vi "mqtt_subsriber.vi"() -> ()   [LabVIEW 2024]
uses:
  <vilib>/LabVIEW Open Source Project/MQTT Client/Client class/Client.lvclass/Client.ctl
  <vilib>/LabVIEW Open Source Project/Connection/Connection.TCP/Connection.TCP.lvclass
  <vilib>/LabVIEW Open Source Project/MQTT Client/Client class/Client.lvclass
  <vilib>/LabVIEW Open Source Project/MQTT Control Packets/Control Packets/PUBLISH/PUBLISH.lvclass
  <vilib>/Utility/file.llb/Write Delimited Spreadsheet (DBL).vi
  <vilib>/LabVIEW Open Source Project/MQTT Connection/MQTT_Base/Base Class/MQTT_Base.lvclass
panel:
  out "Waveform Chart":cluster{"ground_truth":dbl, "predict_flow":dbl}(graph)
  out "String 2":string
  out "String":string
  out "ground_truth":dbl format="%#.1f"
  out "predict_flow":dbl format="%#.1f"
  out "Numeric":i32
  in  "stop":bool
  out "connected":bool
  out "last error":errorcluster
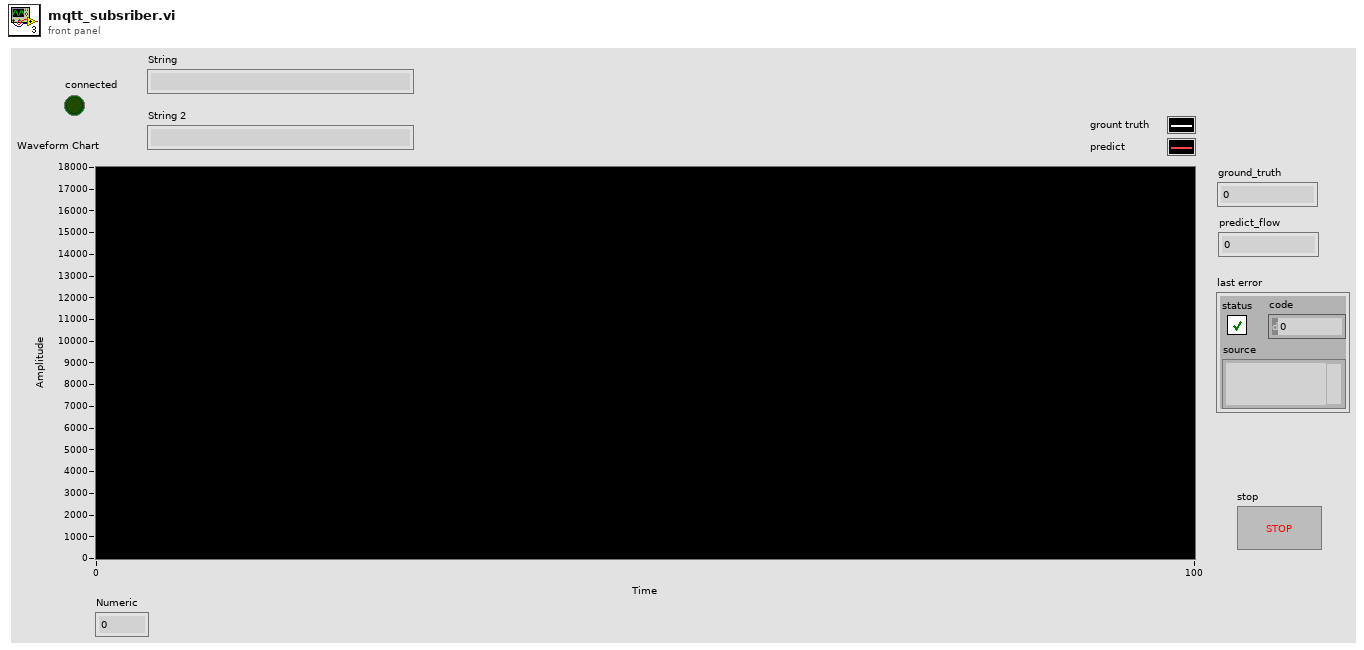
[diagram p1: front panel]
types:
  T1 = typedef "MQTT Client.lvlib/Client.lvclass/Public Events -- cluster.ctl" = cluster{"Connection Status":refnum<user-event>, "Connected":refnum<user-event>, "Application Message":refnum<user-event>}
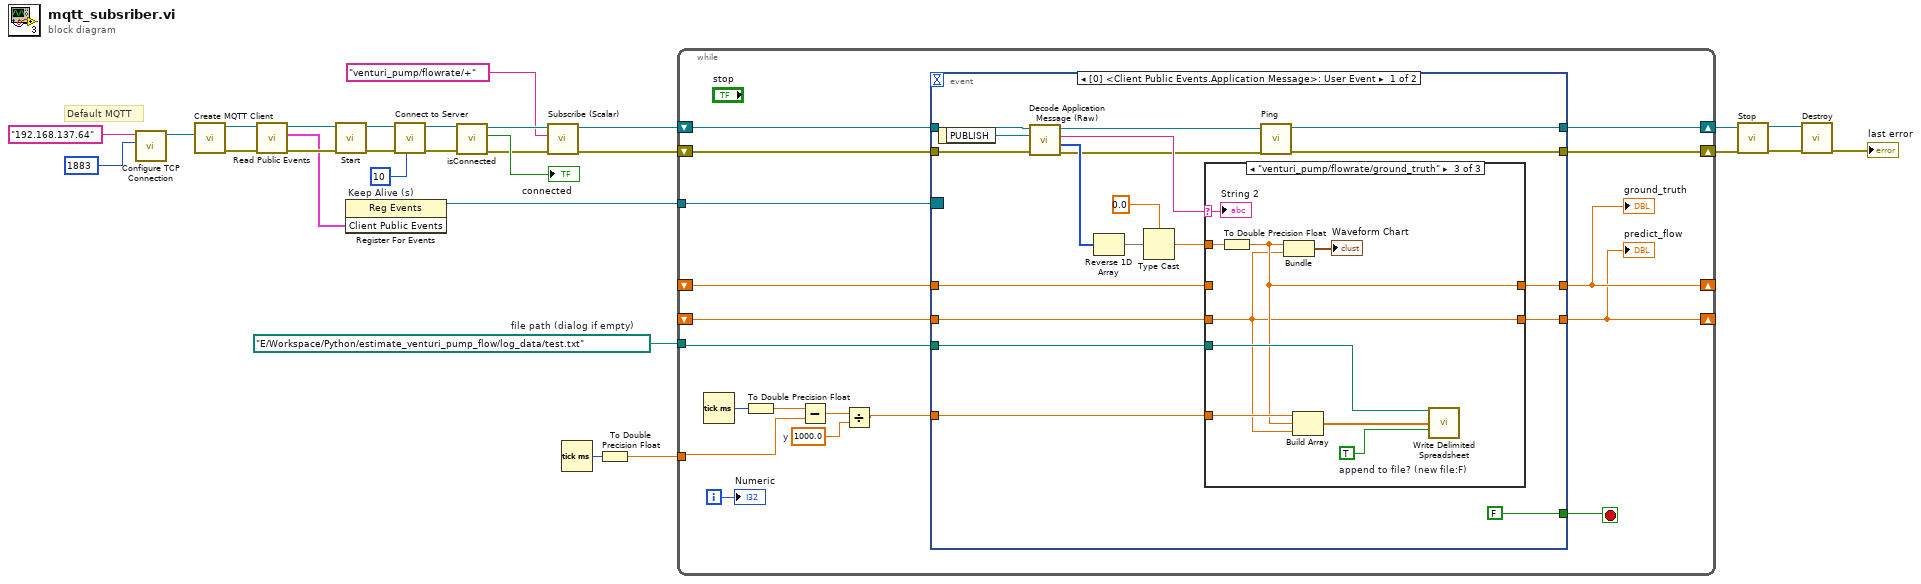
[diagram p0: block diagram]
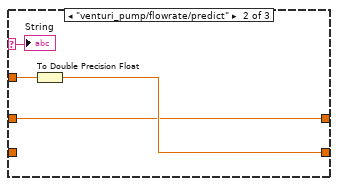
[diagram p3: hidden frame]
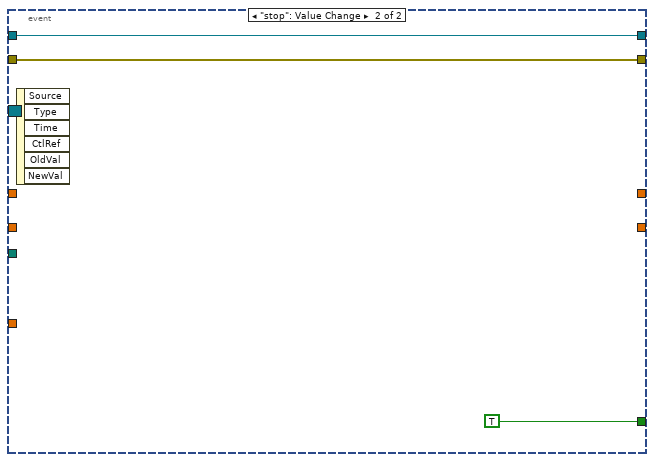
[diagram p4: hidden frame]
diagram:
  w3 = path "E:/Workspace/Python/estimate_venturi_pump_flow/log_data/test.txt"  # file path (dialog if empty)
  w4 = u16 10  # Keep Alive (s)
  # "Default MQTT"
  n1 = call <vilib>:"Configure TCP Connection.vi"("remote port (80)"=u16 1883, "address (localhost)"="192.168.137.64") -> ("Connection.TCP"=w28:refnum<class "Connection.TCP.lvclass">)  [unwired: 8 in, 1 out]
  n2 = call <vilib>:"Create MQTT Client.vi"("Connection Configuration"=w28) -> ("error out"=w14:errorcluster, "Client out"=w15:refnum<class "Client.lvclass">)  [unwired: 9 in]
  n3 = call <vilib>:"Read Public Events.vi"("error in (no error)"=w14, "Client in"=w15) -> ("error out"=w12:errorcluster, "Client Public Events"=w11:T1, "Client out"=w13:refnum<class "Client.lvclass">)  [unwired: 7 in]
  n4 = call <vilib>:"Start.vi"("error in (no error)"=w12, "MQTT_Base in"=w13) -> ("error out"=w18:errorcluster, "MQTT_Base out"=w19:refnum<class "Client.lvclass">)  [unwired: 7 in, 1 out]
  n5 = register-events(w11) -> (reference out=w10:refnum<event-registration>)  [unwired: 2 in, 1 out]
  n6 = call <vilib>:"Connect to Server.vi"("Keep Alive (s)"=w4, "error in (no error)"=w18, "Client in"=w19) -> ("error out"=w16:errorcluster, "Client out"=w17:refnum<class "Client.lvclass">)  [unwired: 5 in, 2 out]
  n7 = call <vilib>:"isConnected.vi"("error in (no error)"=w16, "Client in"=w17) -> ("error out"=w6:errorcluster, "connected"=→"connected":bool, "Client out"=w7:refnum<class "Client.lvclass">)  [unwired: 7 in]
  n8 = call <vilib>:"Subscribe (Scalar).vi"("error in (no error)"=w6, "Topic Filter"="venturi_pump/flowrate/+", "Client in"=w7) -> ("error out"=w8:errorcluster, "Client out"=w9:refnum<class "Client.lvclass">)  [unwired: 6 in, 1 out]
  n9 = Tick Count (ms)() -> (millisecond timer value=w2:u32)
  n10 = To Double Precision Float(number=w2) -> (double precision float=w1:dbl)
  n11 = while {
    shift-right: [w44] -> w22
    shift-left: w9 -> [w46]
    shift-right: [w43] -> w21
    shift-left: w8 -> [w45]
    tunnel: w10 -> [w42]
    tunnel: w3 -> [w29]
    tunnel: w1 -> [w38]
    shift-right: [w32] -> _
    shift-left: _ -> [w34]
    shift-right: [w31] -> _
    shift-left: _ -> [w33]
    i -> [w41]
    stop <- w40 stop-if-true
    w35 = 1000.0  # y
    n12 = Tick Count (ms)() -> (millisecond timer value=w39:u32)
    n13 = To Double Precision Float(number=w39) -> (double precision float=w36:dbl)
    n14 = Subtract(x=w36, y=w38) -> (x-y=w37:dbl)
    n15 = Divide(x=w37, y=w35) -> (x/y=w30:dbl)
    n16 = event shown="[0] <Client Public Events.Application Message>: User Event" {
      selector: w42 -> [_ _]
      dyn-events: _ -> [_ _]
      timeout: _ -> [_ _]
      tunnel: w46 -> [w64 w82]
      tunnel: w45 -> [w63 w81]
      tunnel: [w54 w82] -> w44
      tunnel: [w53 w81] -> w43
      tunnel: [FALSE TRUE] -> w40
      tunnel: [w50 _] -> w32
      tunnel: [w49 _] -> w31
      tunnel: w34 -> [w52 _]
      tunnel: w33 -> [w51 _]
      tunnel: w30 -> [w48 _]
      tunnel: w29 -> [w47 _]
      event User Event {
        n17 = event-data() -> ("PUBLISH"=w61:refnum<class "PUBLISH.lvclass">)  [unwired: 1 in]
        n18 = call <vilib>:"Decode Application Message (Raw).vi"("error in (no error)"=w63, "PUBLISH"=w61, "Client in"=w64) -> ("error out"=w55:errorcluster, "Payload"=w62:u8[], "Topic"=w58:string, "Client out"=w56:refnum<class "Client.lvclass">)  [unwired: 5 in]
        n19 = Reverse 1D Array(array=w62) -> (reversed array=w60:u8[])
        n20 = Type Cast(type=sgl 0.0, x=w60) -> (*(type *) &x=w57:sgl)
        n21 = case shown="\"venturi_pump/flowrate/ground_truth\"" w58 {
          selector: w58 -> [_ w70 w79]
          tunnel: w57 -> [_ w71 w80]
          tunnel: [w67 w68 w73] -> w50
          tunnel: [w66 w69 w72] -> w49
          tunnel: w52 -> [w67 w68 _]
          tunnel: w51 -> [w66 _ w72]
          tunnel: w48 -> [_ _ w76]
          tunnel: w47 -> [_ _ w75]
          frame "False", Default {
          }
          frame "venturi_pump/flowrate/predict" {
            n22 = To Double Precision Float(number=w71) -> (double precision float=w69:dbl)
            "String" <- w70
          }
          frame "venturi_pump/flowrate/ground_truth" {
            w74 = TRUE  # append to file? (new file:F)
            n23 = To Double Precision Float(number=w80) -> (double precision float=w73:dbl)
            n24 = Bundle(w73, w72) -> (→"Waveform Chart":cluster{dbl, dbl})  [unwired: 1 in]
            n25 = Build Array(w76, w73, w72) -> (w78:dbl[])
            n26 = call-poly <vilib>:"Write Delimited Spreadsheet.vi"("file path (dialog if empty)"=w75, "1D data"=w78, "append to file? (new file:F)"=w74) -> ()  [unwired: 11 in, 2 out]
            "String 2" <- w79
          }
        }
        n27 = call <vilib>:"Ping.vi"("error in (no error)"=w55, "Client in"=w56) -> ("error out"=w53:errorcluster, "Client out"=w54:refnum<class "Client.lvclass">)  [unwired: 6 in, 2 out]
      }
      event "stop": Value Change {
        n28 = event-data() -> ()  [unwired: 1 in, 6 out]
      }
    }
    "ground_truth" <- w32
    "predict_flow" <- w31
    "Numeric" <- w41
  }
  n29 = call <vilib>:"Stop.vi"("error in (no error)"=w21, "MQTT_Base in"=w22) -> ("error out"=w26:errorcluster, "MQTT_Base out"=w25:refnum<class "Client.lvclass">)  [unwired: 7 in, 1 out]
  n30 = call <vilib>:"Destroy.vi"("error in (no error)"=w26, "MQTT_Base in"=w25) -> ("error out"=→"last error":errorcluster)  [unwired: 8 in, 1 out]
